vi "Construct.vi"(7 "Use system decimal point (F)":bool, 8 "error in (no error)":errorcluster, 10 "Constants":cluster{"name":string, "value":dbl}[](array[cluster]), 11 "Expression":string) -> (0 "error out":errorcluster, 2 "Variable Names":string[](array[string]), 3 "muExpr out":refnum<class "muExpr.lvclass">)   [LabVIEW 2015, in "muParser.lvlib" / "muExpr.lvclass"]
uses:
  muExpr.lvclass
  muExpr.lvclass/muExpr.ctl
  mupLib/mupCheckError.vi
  <vilib>/Utility/error.llb/Error Cluster From Error Code.vi
  muParser.lvlib
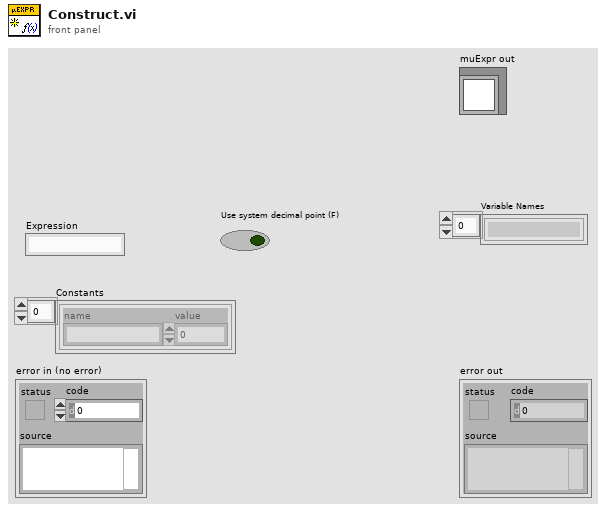
[diagram p1: front panel]
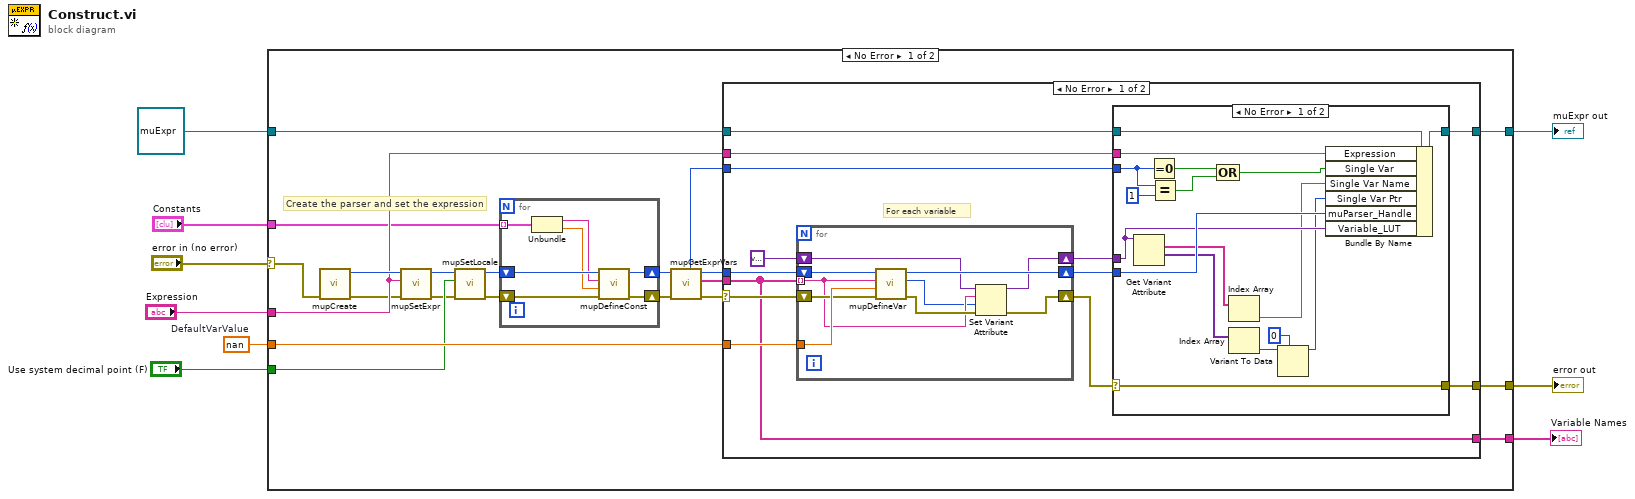
[diagram p0: block diagram]
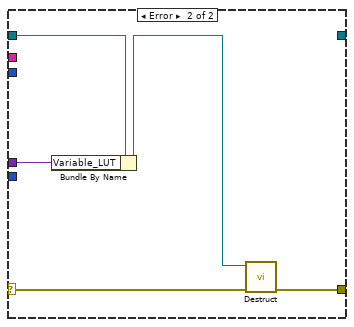
[diagram p2: hidden frame]
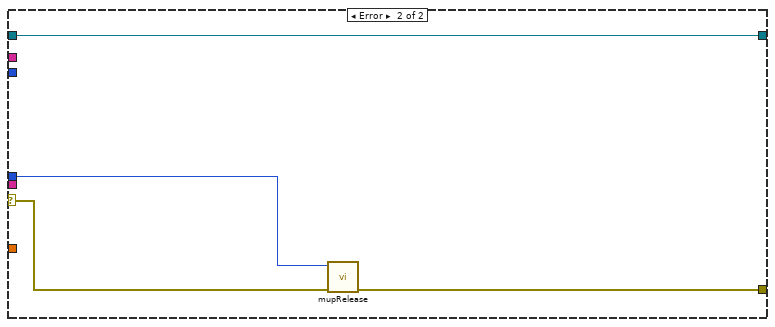
[diagram p3: hidden frame]
diagram:
  w4 = nan  # DefaultVarValue
  n1 = case shown="No Error" "error in (no error)" {
    selector: "error in (no error)" -> [w20 w88]
    tunnel: "Expression" -> [w18 _]
    tunnel: refnum<class "muExpr.lvclass"> refnum ("muExpr out") -> [w30 w87]
    tunnel: [w29 w87] -> w7
    tunnel: [w28 w88] -> w6
    tunnel: w4 -> [w27 _]
    tunnel: [w26 _] -> w3
    tunnel: "Use system decimal point (F)" -> [w21 _]
    tunnel: "Constants" -> [w10 _]
    frame No Error {
      # "Create the parser and set the expression"
      n2 = call "mupCreate.vi"("error in (no error)"=w20) -> ("error out"=w17:errorcluster, "hParser"=w19:u64)  [unwired: 9 in]
      n3 = call "mupSetExpr.vi"("error in (no error)"=w17, "szExpr"=w18, "hParser in"=w19) -> ("error out"=w16:errorcluster, "hParser out"=w15:u64)  [unwired: 7 in]
      n4 = call "mupSetLocale.vi"("error in (no error)"=w16, "Use system decimal point (T)"=w21, "hParser in"=w15) -> ("error out"=w12:errorcluster, "hParser out"=w14:u64)  [unwired: 7 in]
      n5 = for {
        shift-right: [w36] -> w13
        shift-left: w14 -> [w37]
        shift-right: [w34] -> w11
        shift-left: w12 -> [w35]
        tunnel: w10 -> [w33] mode=indexing
        n6 = Unbundle(w33) -> ("name"=w32:string, "value"=w31:dbl)
        n7 = call "mupDefineConst.vi"("error in (no error)"=w35, "Value"=w31, "constName"=w32, "hParser in"=w37) -> ("error out"=w34:errorcluster, "hParser out"=w36:u64)  [unwired: 6 in]
      }
      n8 = call "mupGetExprVars.vi"("error in (no error)"=w11, "hParser in"=w13) -> ("error out"=w24:errorcluster, "varNames"=w23:string[], "hParser out"=w25:u64, "numVars"=w22:i32)  [unwired: 5 in, 1 out]
      n9 = case shown="No Error" w24 {
        selector: w24 -> [w42 w84]
        tunnel: w30 -> [w50 w86]
        tunnel: [w49 w86] -> w29
        tunnel: [w48 w83] -> w28
        tunnel: w22 -> [w46 _]
        tunnel: w27 -> [w43 _]
        tunnel: w25 -> [w44 w85]
        tunnel: w18 -> [w47 _]
        tunnel: [w38 _] -> w26
        tunnel: w23 -> [w38 _]
        frame No Error {
          # "For each variable"
          n10 = for {
            tunnel: w38 -> [w53] mode=indexing
            shift-right: [w54] -> w39
            shift-left: variant -> [w55]
            shift-right: [w59] -> w40
            shift-left: w44 -> [w60]
            tunnel: w43 -> [w58]
            shift-right: [w51] -> w41
            shift-left: w42 -> [w57]
            n11 = call "mupDefineVar.vi"("error in (no error)"=w57, "initValue"=w58, "varName"=w53, "hParser in"=w60) -> ("error out"=w56:errorcluster, "varAddr"=w52:u64, "hParser out"=w59:u64)  [unwired: 5 in]
            n12 = Set Variant Attribute(Variant=w55, name=w53, value=w52, error in=w56) -> (Variant out=w54:variant, error out=w51:errorcluster)  [unwired: 1 out]
          }
          n13 = case shown="No Error" w41 {
            selector: w41 -> [w74 w82]
            tunnel: w50 -> [w77 w80]
            tunnel: [w76 _] -> w49
            tunnel: w40 -> [w75 _]
            tunnel: w39 -> [w72 w78]
            tunnel: [w74 w81] -> w48
            tunnel: w47 -> [w73 _]
            tunnel: w46 -> [w67 _]
            frame No Error {
              n14 = Get Variant Attribute(Variant=w72) -> (names=w71:string[], values=w70:variant[])  [unwired: 3 in, 2 out]
              n15 = Equal To 0?(x=w67) -> (x = 0?=w63:bool)
              n16 = Equal?(x=w67, y=1) -> (x = y?=w62:bool)
              n17 = Compound Arithmetic op=OR(w63, w62) -> (w61:bool)
              n18 = Index Array(array=w71) -> (element=w65:string)  [unwired: 1 in]
              n19 = Index Array(array=w70) -> (element=w69:variant)  [unwired: 1 in]
              n20 = Variant To Data(type=u64 0, Variant=w69) -> (data=w64:u64)  [unwired: 1 in, 1 out]
              n21 = Bundle By Name(cluster=w77, "Expression"=w73, "Single Var"=w61, "Single Var Name"=w65, "Single Var Ptr"=w64, "muParser_Handle"=w75, "Variable_LUT"=w72) -> (w76:refnum<class "muExpr.lvclass">)
            }
            frame Error {
              n22 = Bundle By Name(cluster=w80, "Variable_LUT"=w78) -> (w79:refnum<class "muExpr.lvclass">)
              n23 = call "Destruct.vi"("error in (no error)"=w82, "muExpr in"=w79) -> ("error out"=w81:errorcluster)  [unwired: 9 in]
            }
          }
        }
        frame Error {
          n24 = call "mupRelease.vi"("error in (no error)"=w84, "hParser"=w85) -> ("error out"=w83:errorcluster)  [unwired: 9 in]
        }
      }
    }
    frame Error {
    }
  }
  "error out" <- w6
  "muExpr out" <- w7
  "Variable Names" <- w3
